vi "Asylum_Driver_XYMetersToVoltage.vi"(8 "error in (no error)":errorcluster, 9 "Y Coordinate":dbl, 10 "X Coordinate":dbl, 11 "Application":refnum<k7>) -> (0 "error out":errorcluster, 1 "Y Voltage":dbl, 2 "X Voltage":dbl, 3 "Application":refnum<k7>)   [LabVIEW 2020]
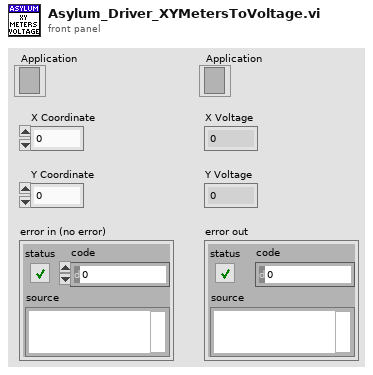
[diagram p1: front panel]
types:
  T1 = cluster{"XLVDT Sens":dbl, "YLVDT Sens":dbl, "XLVDT Offset":dbl, "YLVDT Offset":dbl}
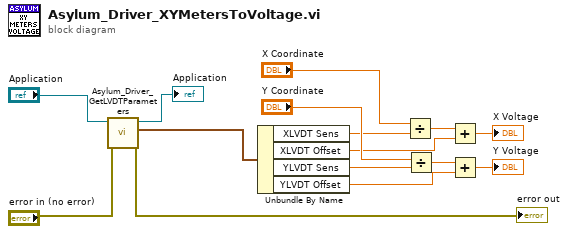
[diagram p0: block diagram]
diagram:
  n1 = call "Asylum_Driver_GetLVDTParameters.vi"("error in (no error)"="error in (no error)", "Application"="Application") -> ("error out"=→"error out":errorcluster, "LVDT Parameters"=w15:T1, "Application"=→"Application":refnum<k7>)  [unwired: 7 in]
  n2 = Unbundle By Name(w15) -> ("XLVDT Sens"=w3:dbl, "XLVDT Offset"=w6:dbl, "YLVDT Sens"=w4:dbl, "YLVDT Offset"=w10:dbl)
  n3 = Divide(x="X Coordinate", y=w3) -> (x/y=w7:dbl)
  n4 = Divide(x="Y Coordinate", y=w4) -> (x/y=w9:dbl)
  n5 = Add(x=w7, y=w6) -> (x+y=→"X Voltage":dbl)
  n6 = Add(x=w9, y=w10) -> (x+y=→"Y Voltage":dbl)
